vi "event_publisher.vi"() -> ()   [LabVIEW 2016]
uses:
  ts_sallv_exa/DataTypes/logevent_SummaryState.ctl
  ts_sallv_exa/DataTypes/logevent_Heartbeat.ctl
  ts_sallv_exa/SALLV_EXA.lvlib
panel:
  in  "Enum":T1(ring)
  out "Stop":bool=TRUE
  in  "stop":bool
  in  "Heartbeat":bool
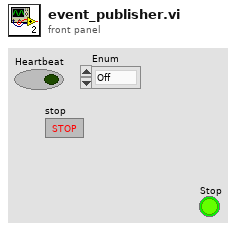
[diagram p1: front panel]
types:
  T1 = enum16{"Off", "Standby", "Enable", "Disable", "Fault"}
  T2 = typedef "SALLV_EXA.lvlib/logevent_SummaryState.ctl" = cluster{"SummaryStateValue":i32, "priority":i32}
  T3 = typedef "SALLV_EXA.lvlib/logevent_Heartbeat.ctl" = cluster{"Heartbeat":bool, "priority":i32}
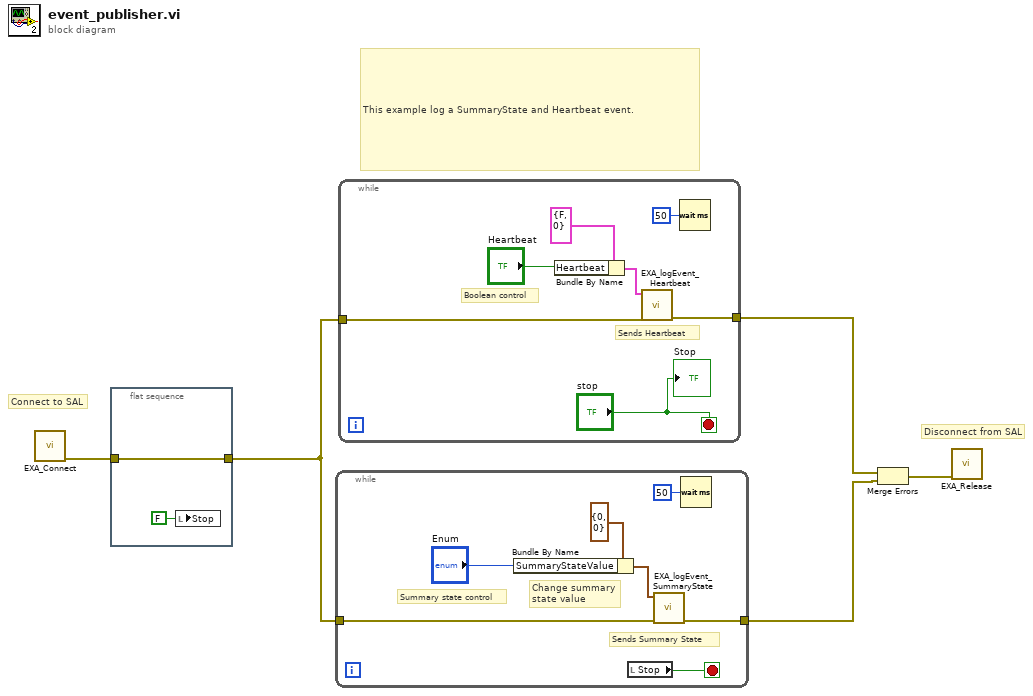
[diagram p0: block diagram]
diagram:
  # "Disconnect from SAL"
  # "Connect to SAL"
  # "This example log a SummaryState and Heartbeat event."
  n1 = call "EXA_Connect.vi"() -> ("error out"=w3:errorcluster)  [unwired: 10 in, 1 out]
  n2 = flat-sequence {
    tunnel: [w7] -> w2
    tunnel: w3 -> [w7]
    frame #0 {
      n3 = local write "Stop"(FALSE ("Stop")) -> ()
    }
  }
  n4 = while {
    tunnel: w2 -> [w12]
    tunnel: [w11] -> w1
    stop <- w14 stop-if-true
    # "Change summary \nstate value"
    # "Summary state control"
    # "Sends Summary State"
    n5 = Bundle By Name(cluster=T2 {"SummaryStateValue"=0, "priority"=0} ("logevent_SummaryState_Ctl"), "SummaryStateValue"="Enum") -> (w8:T2)
    n6 = local read "Stop"() -> (w14:bool)
    n7 = call "EXA_logEvent_SummaryState.vi"("error in (no error)"=w12, "logevent_SummaryState_Ctl"=w8) -> ("error out"=w11:errorcluster)  [unwired: 7 in, 2 out]
    n8 = Wait (ms)(milliseconds to wait=u32 50) -> ()  [unwired: 1 out]
  }
  n9 = while {
    tunnel: w2 -> [w21]
    tunnel: [w17] -> w4
    stop <- "stop" stop-if-true
    # "Boolean control"
    # "Sends Heartbeat"
    n10 = Bundle By Name(cluster=T3 {"Heartbeat"=FALSE, "priority"=0} ("logevent_Heartbeat_Ctl"), "Heartbeat"="Heartbeat") -> (w18:T3)
    n11 = call "EXA_logEvent_Heartbeat.vi"("error in (no error)"=w21, "logevent_Heartbeat_Ctl"=w18) -> ("error out"=w17:errorcluster)  [unwired: 7 in, 2 out]
    n12 = Wait (ms)(milliseconds to wait=u32 50) -> ()  [unwired: 1 out]
    "Stop" <- "stop"
  }
  n13 = Merge Errors(w4, w1) -> (w5:errorcluster)
  n14 = call "EXA_Release.vi"("error in (no error)"=w5) -> ()  [unwired: 9 in, 2 out]
